vi "Avg Temp String Append.vi"(1 "Append String":string=" 1h", 2 "Slave ID":dbl) -> (0 "Avg captions":string[](array[string]))   [LabVIEW 2017, in "GUI.lvlib"]
uses:
  GUI.lvlib
  Konfiguracja/Konfiguracja.lvlib
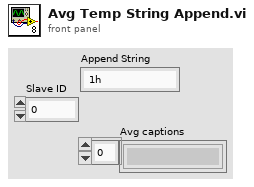
[diagram p1: front panel]
types:
  T1 = cluster{"Termometr 1":string, "Termometr 2":string, "Termometr 3":string, "Termometr 4":string, "Termometr 5":string, "Termometr 6":string, "Termometr 7":string, "Termometr 8":string, "Termometr 9":string, "Termometr 10":string}
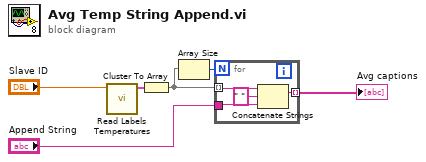
[diagram p0: block diagram]
diagram:
  n1 = call "Read Labels Temperatures.vi"("Slave ID"="Slave ID") -> ("Etykiety T1-10"=w3:T1)  [unwired: 10 in]
  n2 = Cluster To Array(cluster=w3) -> (array=w5:string[])
  n3 = Array Size(array=w5) -> (size(s)=w6:i32)
  n4 = for {
    N: w6 -> [_]
    tunnel: w5 -> [w10] mode=indexing
    tunnel: [w9] -> w2 mode=indexing
    tunnel: "Append String" -> [w8]
    n5 = Concatenate Strings(w10, " " ("string"), w8) -> (w9:string)
  }
  "Avg captions" <- w2
